vi "py-lv-comm_sendCommand.vi"(6 "Wait for response (T)":bool=TRUE, 8 "error in (no error)":errorcluster, 10 "command":string, 11 "zmq_socket in":refnum<class "zmq_socket.lvclass">) -> (0 "error out":errorcluster, 2 "data":string, 3 "zmq_socket out":refnum<class "zmq_socket.lvclass">)   [LabVIEW 2019, in "Sequence Experiment.lvclass"]
doc: "Sends a command via the ZMQ socket.\nIf \"Wait for response\" is False, the function will immediately return after sending. The data string will then be empty.\nIn case \"Wait for response\" is True, the function will block until a message is received on the socket."
uses:
  Sequence Experiment.lvclass
  <vilib>/addons/zeromq/zmq_socket.lvclass
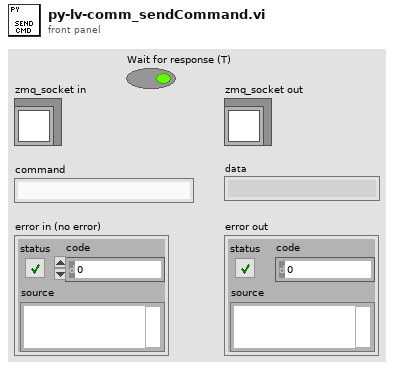
[diagram p1: front panel]
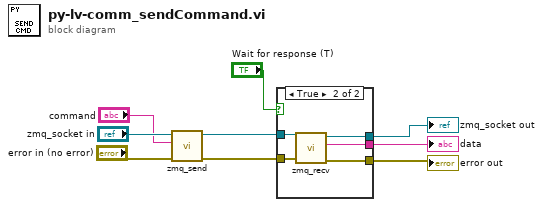
[diagram p0: block diagram]
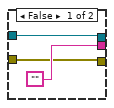
[diagram p2: hidden frame]
diagram:
  n1 = call <vilib>:"zmq_send.vi"("error in"="error in (no error)", "data"="command", "socket in"="zmq_socket in") -> ("error out"=w5:errorcluster, "socket out"=w6:refnum<class "zmq_socket.lvclass">)  [unwired: 4 in]
  n2 = case shown="True" "Wait for response (T)" {
    tunnel: [w11 w15] -> w9
    tunnel: ["" w14] -> w8
    tunnel: [w10 w13] -> w7
    tunnel: w6 -> [w11 w17]
    tunnel: w5 -> [w10 w16]
    frame False {
    }
    frame True {
      n3 = call <vilib>:"zmq_recv.vi"("error in"=w16, "socket in"=w17) -> ("error out"=w13:errorcluster, "data"=w14:string, "socket out"=w15:refnum<class "zmq_socket.lvclass">)  [unwired: 3 in, 2 out]
    }
  }
  "data" <- w8
  "zmq_socket out" <- w9
  "error out" <- w7
